vi "writePos.vi"(1 "Pos":dbl[](array[numeric]), 2 "error in (no error)":errorcluster, 3 "name":string, 4 "ini Path in":path) -> (0 "error out":errorcluster)   [LabVIEW 2016]
uses:
  <vilib>/Utility/config.llb/Write Key (Double).vi
  <vilib>/Utility/config.llb/NI_LVConfig.lvlib
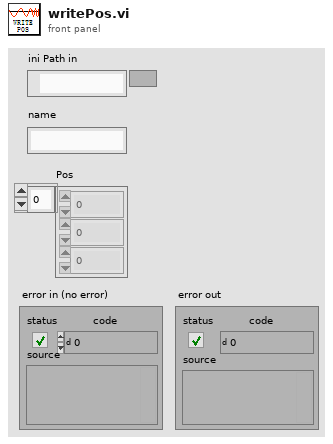
[diagram p1: front panel]
types:
  T1 = typedef "NI_LVConfig.lvlib/Config Data RefNum.ctl" = refnum<k1>
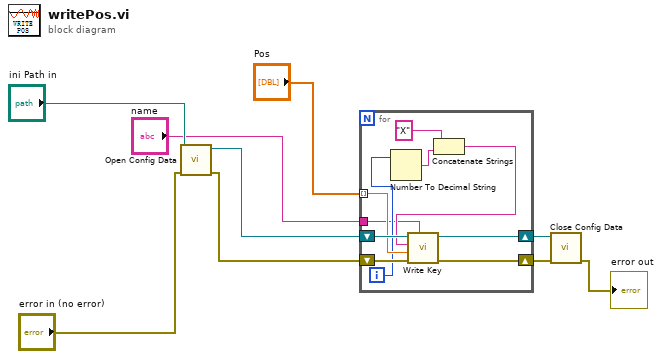
[diagram p0: block diagram]
diagram:
  n1 = call <vilib>:"Open Config Data.vi"("error in (no error)"="error in (no error)", "configuration file path"="ini Path in") -> ("error out"=w6:errorcluster, "refnum"=w5:T1)  [unwired: 7 in, 1 out]
  n2 = for {
    shift-right: [w16] -> w3
    shift-left: w6 -> [w19]
    shift-right: [w17] -> w4
    shift-left: w5 -> [w18]
    tunnel: "Pos" -> [w15] mode=indexing
    tunnel: "name" -> [w10]
    i -> [w14]
    n3 = Number To Decimal String(number=w14) -> (decimal integer string=w12:string)  [unwired: 1 in]
    n4 = Concatenate Strings("X" ("string"), w12) -> (w11:string)
    n5 = call-poly <vilib>:"Write Key.vi"("section"=w10, "error in (no error)"=w19, "value"=w15, "key"=w11, "refnum"=w18) -> ("error out"=w16:errorcluster, "refnum out"=w17:T1)  [unwired: 4 in, 1 out]
  }
  n6 = call <vilib>:"Close Config Data.vi"("error in (no error)"=w3, "refnum"=w4) -> ("error out"=→"error out":errorcluster)  [unwired: 8 in, 1 out]
